vi "View.vi"(8 "error in (no error)":errorcluster, 11 "DAQ View in":refnum<class "DAQ View.lvclass">) -> (0 "error out":errorcluster, 3 "DAQ View out":refnum<class "DAQ View.lvclass">)   [LabVIEW 2022 SP3, in "DAQ View.lvclass"]
uses:
  DAQ View.lvclass
  C:/XY Stage/iView/base view/base view.lvclass
  Accessors/Read DAQ API.lvclass.vi
  iView/base view/Accessors/Read Events.vi
  iView/base view/Accessors/Read View Refnum.vi
  DAQ API/DAQ API.lvclass
  DAQ View.lvclass/DAQ View.ctl
  iView/base view/base view.lvclass
  XY Stage/Process Actor/Process Framework/Process State Data/Process State Data.lvclass
panel:
  out "XY Graph":T1(graph)
  in  "Stop Aquisition":bool
  in  "Aqusition Time":dbl
  in  "Start Button":bool
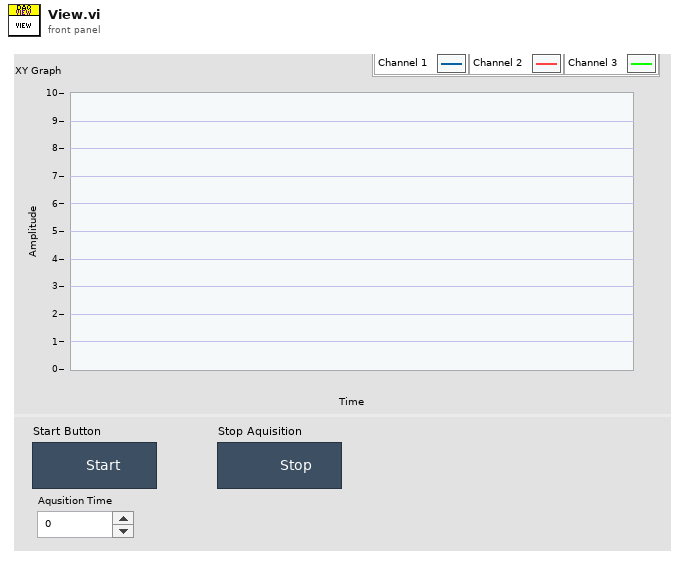
[diagram p1: front panel]
types:
  T1 = cluster{"AI Channel Data":cluster{"Time Stamp":timestamp, "AI":dbl}[]}[]
  T2 = typedef "base view.lvclass/Events.ctl" = cluster{"Open":refnum<user-event>, "Close":refnum<user-event>, "Hide":refnum<user-event>}
  T3 = cluster{"Daq events":refnum<event-registration>, "Process State":refnum<event-registration>, "Event Registration Refnum":refnum<event-registration>}
  T4 = enum8{"Enabled", "Disabled", "Disabled and Grayed Out"}
  T5 = typedef "AI Daq Data.lvlib/AIDAQ Data.ctl" = cluster{"Time Stamp":timestamp, "AI":dbl}
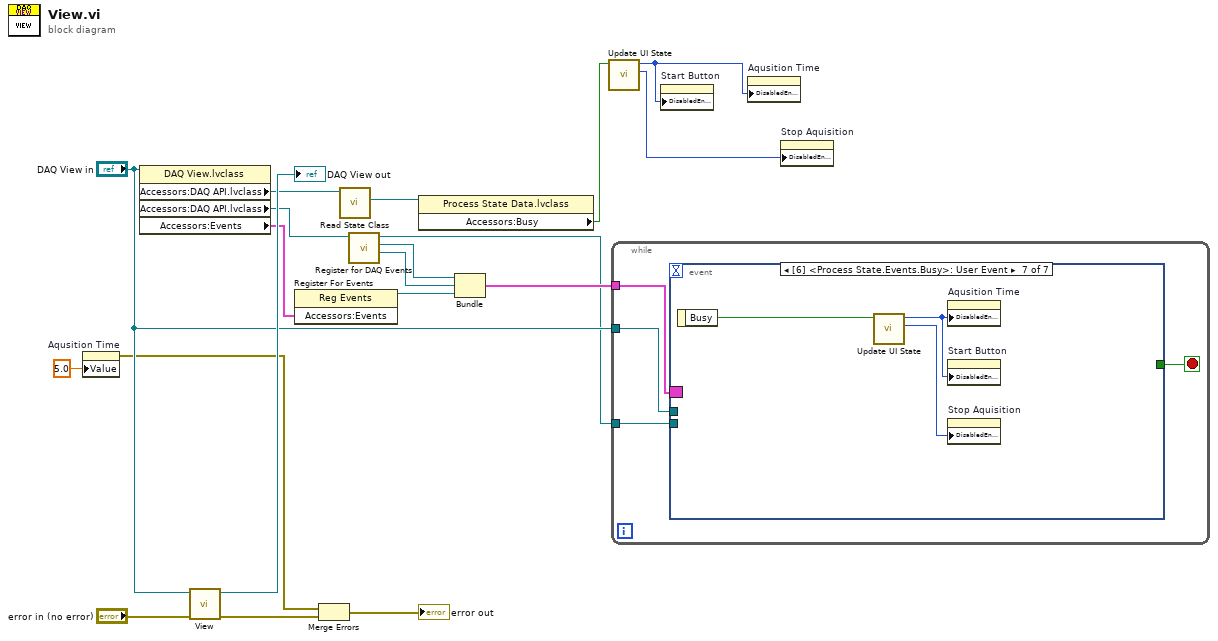
[diagram p0: block diagram]
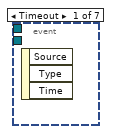
[diagram p2: hidden frame]
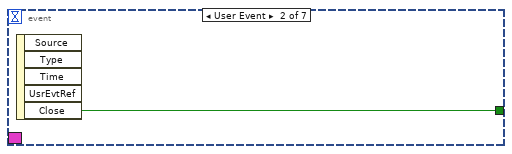
[diagram p3: hidden frame]
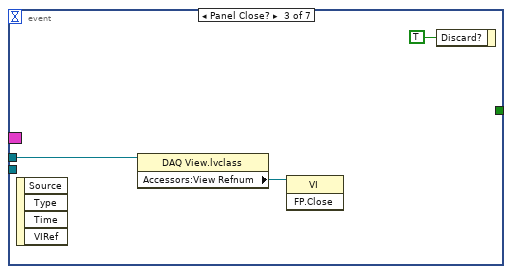
[diagram p4: hidden frame]
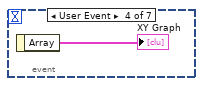
[diagram p5: hidden frame]
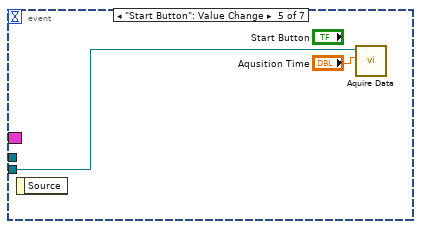
[diagram p6: hidden frame]
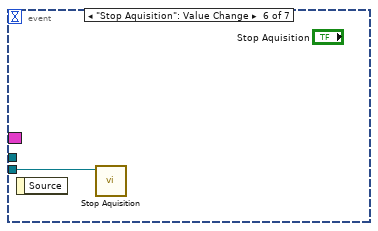
[diagram p7: hidden frame]
diagram:
  n1 = property on="Aqusition Time" class="DigNum (strict)"("Value"=5.0 ("Aqusition Time")) -> (error out=w8:errorcluster)  [unwired: 2 in, 1 out]
  n2 = property class="DAQ View.lvclass"(reference="DAQ View in") -> ("Accessors:DAQ API.lvclass"=w5:refnum<class "DAQ API.lvclass">, "Accessors:DAQ API.lvclass"=w15:refnum<class "DAQ API.lvclass">, "Accessors:Events"=w16:T2)  [unwired: 1 in, 2 out]
  n3 = call-parent "View.vi"("error in (no error)"="error in (no error)", "base view in"="DAQ View in") -> ("error out"=w6:errorcluster, "base view out"=→"DAQ View out":refnum<class "DAQ View.lvclass">)  [unwired: 8 in]
  n4 = register-events(w16) -> (reference out=w17:refnum<event-registration>)  [unwired: 2 in, 1 out]
  n5 = Merge Errors(w8, w6) -> (→"error out":errorcluster)
  n6 = call-dynamic "Read State Class.vi"("Get Daq Status in"=w5) -> ("Process State Data"=w4:refnum<data-value>)  [unwired: 8 in, 2 out]
  n7 = call-dynamic "Register for DAQ Events.vi"("Get Daq Status in"=w15) -> ("Process State"=w13:refnum<event-registration>, "Daq events"=w12:refnum<event-registration>, "Get Daq Status out"=w10:refnum<class "DAQ API.lvclass">)  [unwired: 7 in, 1 out]
  n8 = property class="Process State Data.lvclass"(reference=w4) -> ("Accessors:Busy"=w3:bool)  [unwired: 1 in, 2 out]
  n9 = Bundle("Daq events"=w12, "Process State"=w13, "Event Registration Refnum"=w17) -> (w14:T3)  [unwired: 1 in]
  n10 = call "Update UI State.vi"("Busy"=w3) -> ("Disabled 2"=w1:T4, "Disabled"=w2:T4)  [unwired: 9 in]
  n11 = while {
    tunnel: w14 -> [w23]
    tunnel: "DAQ View in" -> [w21]
    tunnel: w10 -> [w20]
    stop <- w22 stop-if-true
    n12 = event shown="[6] <Process State.Events.Busy>: User Event" {
      selector: w23 -> [_ _ _ _ _ _ _]
      dyn-events: _ -> [_ _ _ _ _ _ _]
      timeout: _ -> [_ _ _ _ _ _ _]
      tunnel: [_ w24 _ _ _ _ _] -> w22
      tunnel: w21 -> [_ _ w25 _ _ _ _]
      tunnel: w20 -> [_ _ _ _ w30 w31 _]
      event Timeout {
        n13 = event-data() -> ()  [unwired: 1 in, 3 out]
      }
      event User Event {
        n14 = event-data() -> ("Close"=w24:bool)  [unwired: 1 in, 4 out]
      }
      event Panel Close? {
        n15 = event-data() -> ()  [unwired: 1 in, 4 out]
        n16 = property class="DAQ View.lvclass"(reference=w25) -> ("Accessors:View Refnum"=w27:refnum<vi>)  [unwired: 1 in, 2 out]
        n17 = invoke class="VI" method="FP.Close"(reference=w27) -> ()  [unwired: 2 in, 3 out]
        n18 = event-data("Discard?"=TRUE) -> ()  [unwired: 1 in, 1 out]
      }
      event User Event {
        n19 = event-data() -> ("Array"=→"XY Graph":cluster{"AI Channel Data":T5[]}[])  [unwired: 1 in]
      }
      event "Start Button": Value Change {
        n20 = event-data() -> ()  [unwired: 1 in, 1 out]
        n21 = call-dynamic "Aquire Data.vi"("Aqusition Time (s)"="Aqusition Time", "Aquire Data in"=w30) -> ()  [unwired: 8 in, 2 out]
      }
      event "Stop Aquisition": Value Change {
        n22 = event-data() -> ()  [unwired: 1 in, 1 out]
        n23 = call-dynamic "Stop Aquisition.vi"("Aquire Data in"=w31) -> ()  [unwired: 9 in, 2 out]
      }
      event User Event {
        n24 = event-data() -> ("Busy"=w34:bool)  [unwired: 1 in]
        n25 = call "Update UI State.vi"("Busy"=w34) -> ("Disabled 2"=w33:T4, "Disabled"=w32:T4)  [unwired: 9 in]
        n26 = property on="Aqusition Time" class="DigNum (strict)"("DisabledEnum"=w32) -> ()  [unwired: 2 in, 2 out]
        n27 = property on="Start Button" class="Bool"("DisabledEnum"=w32) -> ()  [unwired: 2 in, 2 out]
        n28 = property on="Stop Aquisition" class="Bool"("DisabledEnum"=w33) -> ()  [unwired: 2 in, 2 out]
      }
    }
  }
  n29 = property on="Start Button" class="Bool"("DisabledEnum"=w2) -> ()  [unwired: 2 in, 2 out]
  n30 = property on="Aqusition Time" class="DigNum (strict)"("DisabledEnum"=w2) -> ()  [unwired: 2 in, 2 out]
  n31 = property on="Stop Aquisition" class="Bool"("DisabledEnum"=w1) -> ()  [unwired: 2 in, 2 out]
